vi "FileTransferOptionsToRef.vi"(8 "error in (no error)":errorcluster, 10 "FileTransferOptions":refnum<class "FileTransferOptions.lvclass">, 11 "FileTransfer in":refnum<class "FileTransfer.lvclass">) -> (0 "error out":errorcluster, 2 "TransferOptions Ref":refnum<k24>)   [LabVIEW 2015, in "WinSCP.lvlib" / "FileTransfer.lvclass"]
uses:
  FileTransfer.lvclass
  FileTransferOptions/FileTransferOptions.lvclass
  C:/Users/Public/Documents/Projects/lv-winscp/Bin WinSCP/WinSCPnet.dll
  Bin WinSCP/WinSCPnet.dll
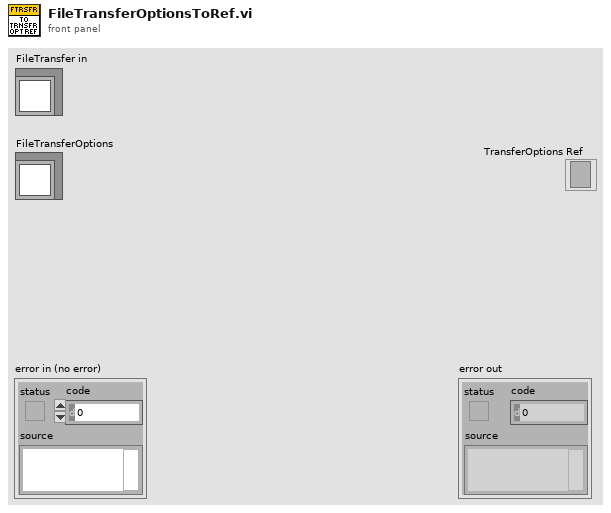
[diagram p1: front panel]
types:
  T1 = typedef "WinSCP.lvlib/FileTransferOptions.lvclass/TransferMode.ctl" = enum16{"Binary", "Ascii", "Auto"}
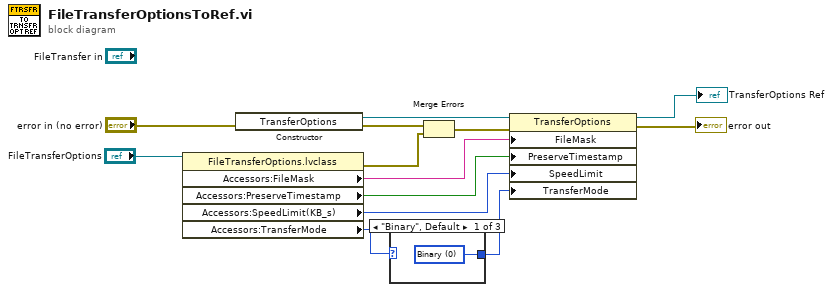
[diagram p0: block diagram]
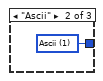
[diagram p2: hidden frame]
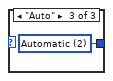
[diagram p3: hidden frame]
diagram:
  n1 = property class="FileTransferOptions.lvclass"(reference="FileTransferOptions") -> (error out=w8:errorcluster, "Accessors:FileMask"=w7:string, "Accessors:PreserveTimestamp"=w6:bool, "Accessors:SpeedLimit(KB_s)"=w5:i32, "Accessors:TransferMode"=w3:T1)  [unwired: 1 in, 1 out]
  n2 = constructor class="TransferOptions"(error in="error in (no error)") -> (reference out=w11:refnum<k24>, error out=w10:errorcluster)  [unwired: 2 in, 1 out]
  n3 = case shown="\"Binary\", Default" w3 {
    tunnel: [w14 w15 w16] -> w4
    frame "Binary", Default {
      w14 = 0 items=["Binary", "Ascii", "Automatic"] ("TransferMode")
    }
    frame "Ascii" {
      w15 = 1 items=["Binary", "Ascii", "Automatic"] ("TransferMode")
    }
    frame "Auto" {
      w16 = 2 items=["Binary", "Ascii", "Automatic"] ("TransferMode")
    }
  }
  n4 = Merge Errors(w10, w8) -> (w9:errorcluster)
  n5 = property class="TransferOptions"(reference=w11, error in=w9, "FileMask"=w7, "PreserveTimestamp"=w6, "SpeedLimit"=w5, "TransferMode"=w4) -> (reference out=→"TransferOptions Ref":refnum<k24>, error out=→"error out":errorcluster)
